vi "Main.vi"(8 "error in (no error)":errorcluster, 11 "wavefront sensorBase in":refnum<class "wavefront sensor.lvclass">) -> (0 "error out":errorcluster, 3 "component":refnum<class "wavefront sensor.lvclass">)   [LabVIEW 2012, in "wavefront sensor.lvclass"]
doc: "Main VI of the component."
uses:
  wavefront sensor.lvclass
  <vilib>/Distrio/Murmex/Murmex/command_enum.ctl
  <vilib>/Distrio/Murmex/InitialiseMessage/InitialiseMessage.lvclass
  <vilib>/Distrio/Murmex/TerminateMessage/TerminateMessage.lvclass
  <vilib>/Distrio/Murmex/ConfigureMessage/ConfigureMessage.lvclass
  <vilib>/Distrio/Murmex/Murmex/Set configure at initialise.vi
  <vilib>/Distrio/Murmex/Murmex/Set log reference.vi
  <vilib>/Distrio/Murmex/Murmex/Set VI reference.vi
  <vilib>/Distrio/Murmex/Murmex/Get ID.vi
  <vilib>/Distrio/Murmex/Murmex/Murmex.lvclass
  <vilib>/Distrio/Murmex/Message/Message.lvclass
panel:
  in  "Tab Control":enum32{"Page 1", "Page 2"}(tab)
  in  "button:configure":bool
  in  "command":T1
  in  "generic command":string
  in  "button:send command":bool
  in  "button:quit":bool
  out "terminate?":bool
  out "log":string
  in  "Component id":string="BMC"
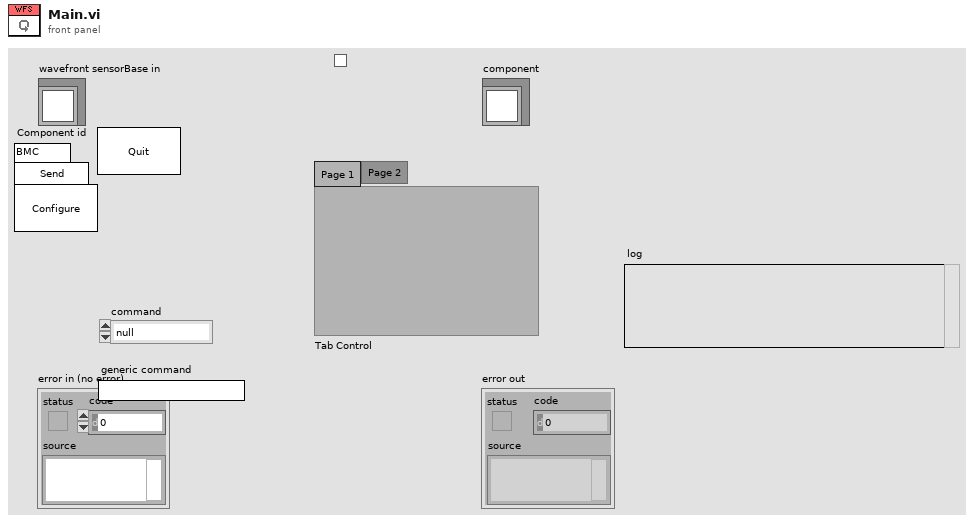
[diagram p1: front panel]
types:
  T1 = typedef "Murmex.lvlib/Murmex.lvclass/command_enum.ctl" = enum16{"null", "initialise", "reset", "terminate", "acknowledge", "update", "inspect", "inform", "proceed", "start", "stop", "fetch", "configure", "generic"}
  T2 = enum8{"Enabled", "Disabled", "Disabled and Grayed Out"}
  T3 = typedef "Murmex.lvclass/command_enum.ctl" = enum16{"null", "initialise", "reset", "terminate", "acknowledge", "update", "inspect", "inform", "proceed", "start", "stop", "fetch", "configure", "generic"}
  T4 = typedef "Murmex.lvclass/Event type enumerations.ctl" = enum16{"before", "after"}
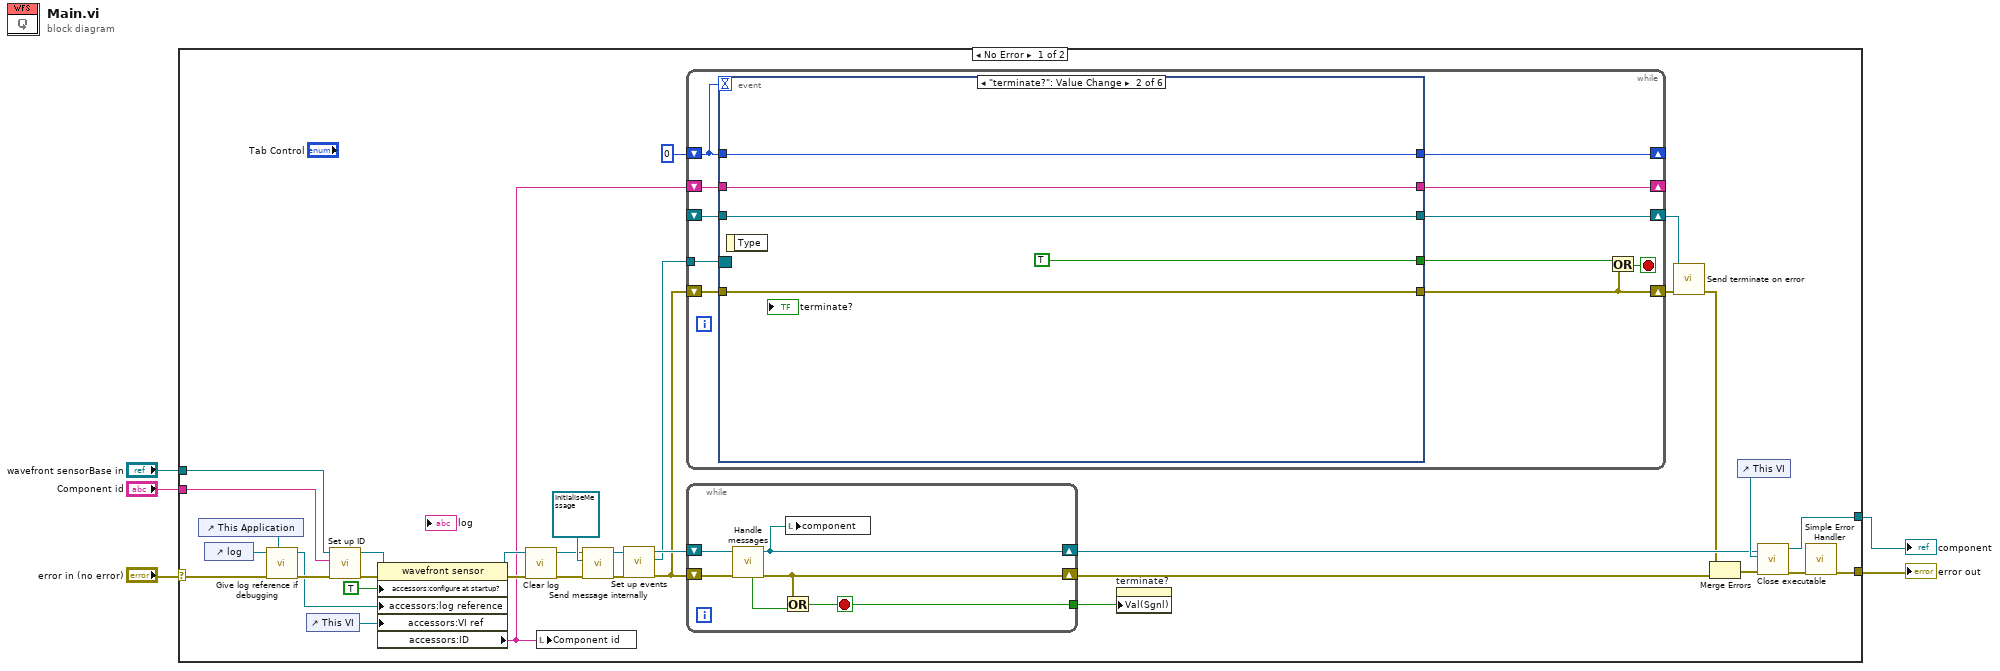
[diagram p0: block diagram]
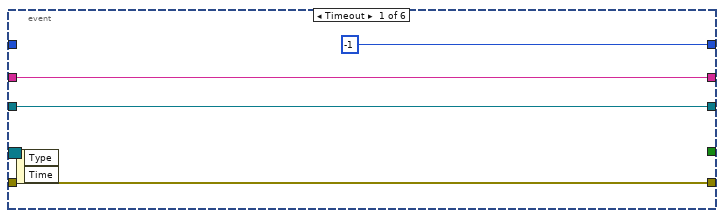
[diagram p2: hidden frame]
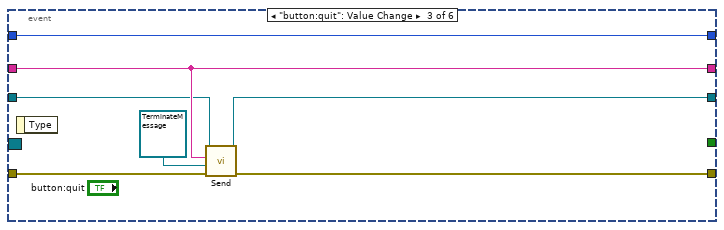
[diagram p3: hidden frame]
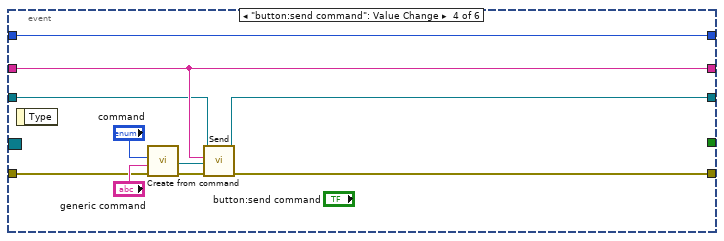
[diagram p4: hidden frame]
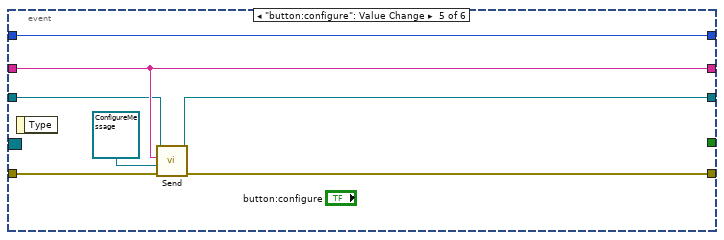
[diagram p5: hidden frame]
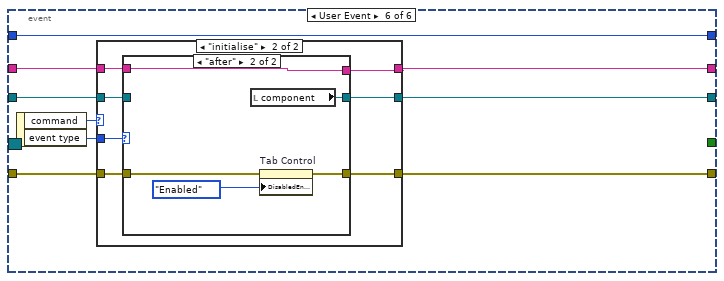
[diagram p6: hidden frame]
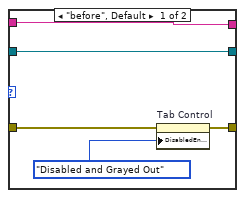
[diagram p8: hidden frame]
diagram:
  n1 = case shown="No Error" "error in (no error)" {
    selector: "error in (no error)" -> [w36 w120]
    tunnel: "wavefront sensorBase in" -> [w35 w119]
    tunnel: "Component id" -> [w34 _]
    tunnel: [w15 w120] -> w2
    tunnel: [w14 w119] -> w1
    frame No Error {
      n2 = control-ref of="This Application"() -> (w37:refnum<vi>)
      n3 = control-ref of="log"() -> (w38:refnum<vi>)
      n4 = call "Give log reference if debugging.vi"("application ref"=w37, "error in (no error)"=w36, "log reference in"=w38) -> ("error out"=w39:errorcluster, "log reference out"=w30:refnum<vi>)  [unwired: 6 in, 1 out]
      n5 = control-ref of="This VI"() -> (w29:refnum<vi>)
      n6 = call <vilib>:"Set up ID.vi"("error in (no error)"=w39, "component ID"=w34, "MurmexBase in"=w35) -> ("error out"=w33:errorcluster, "MurmexBase out"=w32:refnum<class "wavefront sensor.lvclass">)  [unwired: 6 in, 1 out]
      n7 = property class="wavefront sensor"(reference=w32, error in=w33, "accessors:configure at startup?"=TRUE ("configure at startup?"), "accessors:log reference"=w30, "accessors:VI ref"=w29) -> (reference out=w22:refnum<class "wavefront sensor.lvclass">, error out=w23:errorcluster, "accessors:ID"=w10:string)
      n8 = call <vilib>:"Clear log.vi"("error in (no error)"=w23, "MurmexBase in"=w22) -> ("error out"=w25:errorcluster, "MurmexBase out"=w24:refnum<class "wavefront sensor.lvclass">)  [unwired: 8 in]
      n9 = local write "Component id"(w10) -> ()
      n10 = call <vilib>:"Send message internally.vi"("error in (no error)"=w25, "Message"=refnum<class "InitialiseMessage.lvclass"> refnum ("InitialiseMessage"), "Murmex in"=w24) -> ("error out"=w27:errorcluster, "Murmex out"=w28:refnum<class "wavefront sensor.lvclass">)  [unwired: 7 in]
      n11 = call <vilib>:"Set up events.vi"("error in (no error)"=w27, "MurmexBase in"=w28) -> ("error out"=w11:errorcluster, "Event Registration Refnum"=w12:refnum<event-registration>, "MurmexBase out"=w21:refnum<class "wavefront sensor.lvclass">)  [unwired: 7 in]
      n12 = while {
        tunnel: w12 -> [w42]
        shift-right: [w44] -> w8
        shift-left: w11 -> [w46]
        shift-right: [w47] -> _
        shift-left: w10 -> [w48]
        shift-right: [w49] -> _
        shift-left: 0 -> [w50]
        shift-right: [w41] -> w6
        shift-left: _ -> [w40]
        stop <- w45 stop-if-true
        n13 = event shown="[1] \"terminate?\": Value Change" {
          selector: w42 -> [_ _ _ _ _ _]
          dyn-events: _ -> [_ _ _ _ _ _]
          timeout: w50 -> [_ _ _ _ _ _]
          tunnel: w50 -> [_ w56 w62 w69 w80 w92]
          tunnel: [-1 w56 w62 w69 w80 w92] -> w49
          tunnel: w48 -> [w53 w57 w63 w70 w79 w89]
          tunnel: [w53 w57 w63 w70 w79 w88] -> w47
          tunnel: w46 -> [w52 w59 w66 w72 w82 w87]
          tunnel: [w52 w59 w65 w71 w81 w86] -> w44
          tunnel: [_ TRUE _ _ _ _] -> w43
          tunnel: [w51 w55 w60 w67 w77 w91] -> w41
          tunnel: w40 -> [w51 w55 w61 w68 w78 w90]
          event Timeout {
            n14 = event-data() -> ()  [unwired: 1 in, 2 out]
          }
          event "terminate?": Value Change {
            n15 = event-data() -> ()  [unwired: 1 in, 1 out]
          }
          event "button:quit": Value Change {
            n16 = event-data() -> ()  [unwired: 1 in, 1 out]
            n17 = call <vilib>:"Send.vi"("error in (no error)"=w66, "Message"=refnum<class "TerminateMessage.lvclass"> refnum ("TerminateMessage"), "recipient"=w63, "Murmex in"=w61) -> ("error out"=w65:errorcluster, "Murmex out"=w60:refnum<class "wavefront sensor.lvclass">)  [unwired: 6 in]
          }
          event "button:send command": Value Change {
            n18 = event-data() -> ()  [unwired: 1 in, 1 out]
            n19 = call <vilib>:"Create from command.vi"("error in (no error)"=w72, "generic command"="generic command", "command"="command") -> ("error out"=w76:errorcluster, "Message out"=w73:refnum<class "Message.lvclass">)  [unwired: 7 in]
            n20 = call <vilib>:"Send.vi"("error in (no error)"=w76, "Message"=w73, "recipient"=w70, "Murmex in"=w68) -> ("error out"=w71:errorcluster, "Murmex out"=w67:refnum<class "wavefront sensor.lvclass">)  [unwired: 6 in]
          }
          event "button:configure": Value Change {
            n21 = event-data() -> ()  [unwired: 1 in, 1 out]
            n22 = call <vilib>:"Send.vi"("error in (no error)"=w82, "Message"=refnum<class "ConfigureMessage.lvclass"> refnum ("ConfigureMessage"), "recipient"=w79, "Murmex in"=w78) -> ("error out"=w81:errorcluster, "Murmex out"=w77:refnum<class "wavefront sensor.lvclass">)  [unwired: 6 in]
          }
          event User Event {
            n23 = event-data() -> ("command"=w85:T3, "event type"=w84:T4)  [unwired: 1 in]
            n24 = case shown="\"initialise\"" w85 {
              tunnel: w84 -> [_ w102]
              tunnel: w87 -> [w93 w101]
              tunnel: w89 -> [w94 w100]
              tunnel: [w94 w99] -> w88
              tunnel: [w95 w98] -> w91
              tunnel: w90 -> [w95 w97]
              tunnel: [w93 w96] -> w86
              frame "null", Default {
              }
              frame "initialise" {
                n25 = case shown="\"after\"" w102 {
                  tunnel: w101 -> [w104 w112]
                  tunnel: [w103 w110] -> w96
                  tunnel: [w106 w108] -> w99
                  tunnel: w100 -> [w106 w108]
                  tunnel: [w107 w109] -> w98
                  tunnel: w97 -> [w107 _]
                  frame "before", Default {
                    n26 = property on="Tab Control" class="TabCtl (strict)"(error in=w104, "DisabledEnum"=T2."Disabled and Grayed Out" ("Disabled")) -> (error out=w103:errorcluster)  [unwired: 1 in, 1 out]
                  }
                  frame "after" {
                    n27 = local read "component"() -> (w109:refnum<class "wavefront sensor.lvclass">)
                    n28 = property on="Tab Control" class="TabCtl (strict)"(error in=w112, "DisabledEnum"=T2."Enabled" ("Disabled")) -> (error out=w110:errorcluster)  [unwired: 1 in, 1 out]
                  }
                }
              }
            }
          }
        }
        n29 = Or(x=w43, y=w44) -> (x .or. y?=w45:bool)
      }
      n30 = while {
        shift-right: [w116] -> w16
        shift-left: w21 -> [w117]
        shift-right: [w115] -> w17
        shift-left: w11 -> [w118]
        tunnel: [w113] -> w13
        stop <- w113 stop-if-true
        n31 = call <vilib>:"Handle messages.vi"("error in (no error)"=w118, "Murmex in"=w117) -> ("error out"=w115:errorcluster, "Murmex out"=w116:refnum<class "wavefront sensor.lvclass">, "terminated?"=w114:bool)  [unwired: 7 in]
        n32 = Or(x=w115, y=w114) -> (x .or. y?=w113:bool)
        n33 = local write "component"(w116) -> ()
      }
      n34 = property on="terminate?" class="Bool (strict)"("Val(Sgnl)"=w13) -> ()  [unwired: 2 in, 2 out]
      n35 = call <vilib>:"Send terminate on error.vi"("error in (no error)"=w8, "Murmex in"=w6) -> ("error out"=w7:errorcluster)  [unwired: 8 in, 1 out]
      n36 = Merge Errors(w7, w17) -> (w19:errorcluster)
      n37 = control-ref of="This VI"() -> (w20:refnum<vi>)
      n38 = call <vilib>:"Close executable.vi"("error in (no error)"=w19, "main VI ref (optional)"=w20, "MurmexBase in"=w16) -> ("error out"=w18:errorcluster, "MurmexBase out"=w14:refnum<class "wavefront sensor.lvclass">)  [unwired: 7 in]
      n39 = call <vilib>:"Simple Error Handler.vi"("error in (no error)"=w18) -> ("error out"=w15:errorcluster)  [unwired: 4 in, 4 out]
    }
    frame Error {
    }
  }
  "error out" <- w2
  "component" <- w1
